vi "Register Status Change Event.vi"() -> ()   [LabVIEW 2017]
doc: "------------- lvcsm -------------\n[CSMStates]\nItem 0 = \"Event Structure\"\nItem 1 = \"Idle\"\nItem 2 = \"CSM Documentation\"\nItem 3 = \"VI Reference\"\nItem 4 = \"Error Handler\"\nItem 5 = \"Critical Error\"\nItem 6 = \"Target Timeout Error\"\nItem 7 = \"Target Error\"\nItem 8 = \"Async Response\"\nItem 9 = \"Response\"\nItem 10 = \"Async Message Posted\"\nItem 11 = \"Initialize Core Data\"\nItem 12 = \"Exit\"\nItem 13 = \"Data: Initialize\"\nItem 14 = \"Data: Cleanup\"\nItem 15 = \"Events: Register\"\nItem 16 = \"Events: Unregister\"\nItem 17 = \"UI: Initialize\"\nItem 18 = \"UI: Cursor Set\"\nItem 19 = \"UI: Front Panel State\"\nItem 20 = \"Macro: Initialize\"\nItem 21 = \"Macro: Exit\"\nItem 22 = \"API: API1\"\nItem 23 = \"API: API2\"\nItem 24 = \"DoSth: DoA\"\nItem 25 = \"DoSth: DoB\"\nItem 26 = \"Handler: Error Occurred\"\n\n[CSMStatus]\nItem 0 = \"Error Occured@\"\nItem 1 = \"Slave Status Changed@\"\nItem 2 = \"Slave Status Changed@\""
uses:
  user.lib/_NEVSTOP/Communicable State Machine(CSM)/AdvanceAPI/CSM - Revert Arguments-Safe String.vi
  user.lib/_NEVSTOP/Communicable State Machine(CSM)/AdvanceAPI/CSM - Break Down Multiple States String.vi
  user.lib/_NEVSTOP/Communicable State Machine(CSM)/AdvanceAPI/CSM - Compact Multiple States.vi
  user.lib/_NEVSTOP/Communicable State Machine(CSM)/AdvanceAPI/CSM - Make String Arguments Safe.vi
  user.lib/_NEVSTOP/Communicable State Machine(CSM)/AdvanceAPI/CSM - Keywords.vi
  user.lib/_NEVSTOP/Communicable State Machine(CSM)/_Shared/Trim Single-line Text.vi
  user.lib/_NEVSTOP/Communicable State Machine(CSM)/_Polymophic/Build Unregister Message.vi
  user.lib/_NEVSTOP/Communicable State Machine(CSM)/_Polymophic/Build Register Message.vi
  user.lib/_NEVSTOP/Communicable State Machine(CSM)/Communicable State Machine.lvlib
panel:
  in  "unregister":bool
  in  "register":bool
  in  "empty":bool
  in  "simulate an error":bool
  in  "Status Change":bool
  out "State History 2":string
  out "State History":string
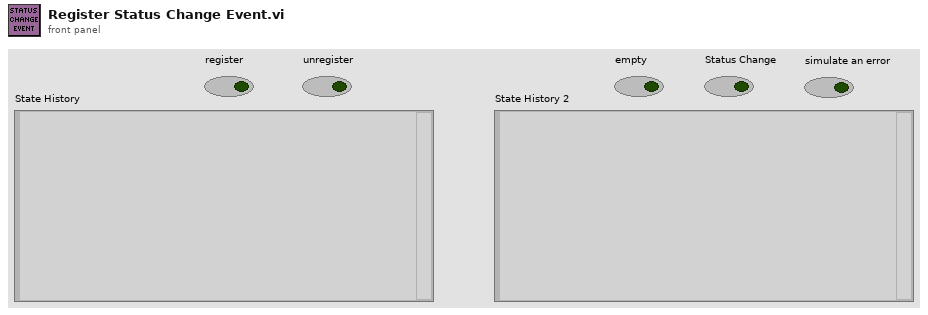
[diagram p1: front panel]
types:
  T1 = enum32{"Invalid", "Standard", "Closed", "Hidden", "Minimized", "Maximized"}
  T2 = enum32{"invalid app kind", "Development System", "Run Time System", "Student Edition", "Embedded LabVIEW", "Evaluation", "Custom"}
  T3 = typedef "Communicable State Machine.lvlib/_CSM_Response Source Message.ctl" = cluster{"‘State":string, "’Arguments":string, "’Error":errorcluster}
  T4 = cluster{"Current VI Reference":refnum<vi>, "Close Panel on Exit?":bool}
  T5 = cluster{"Core":cluster{"Current VI Reference":refnum<vi>, "Close Panel on Exit?":bool}, "Your Boolean data":bool, "Your string data":string}
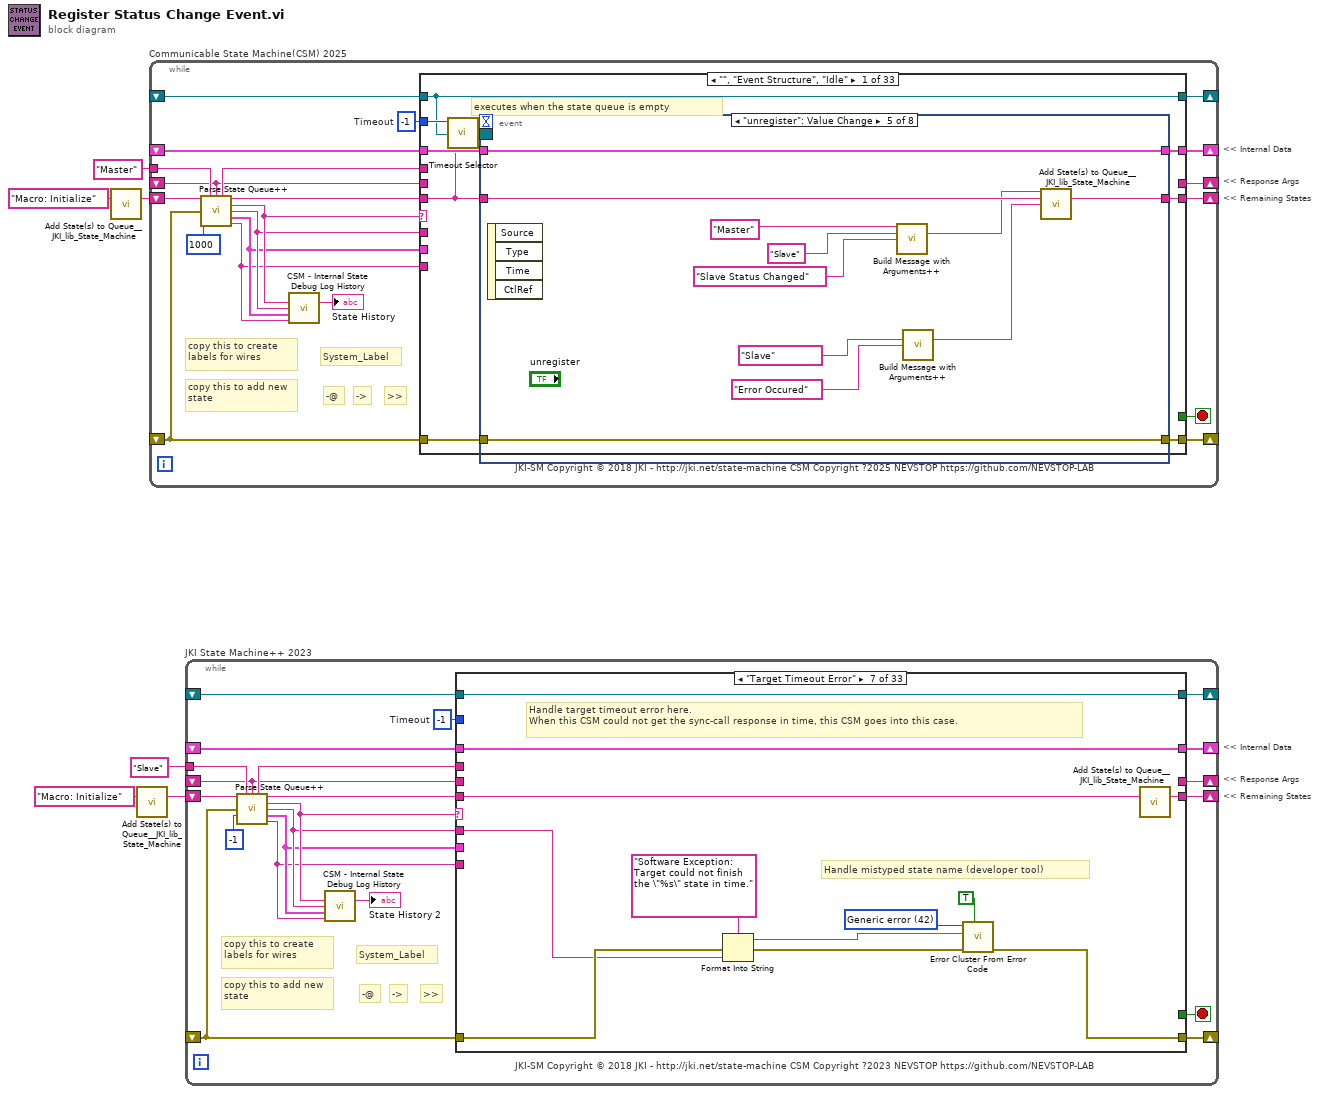
[diagram p0: block diagram]
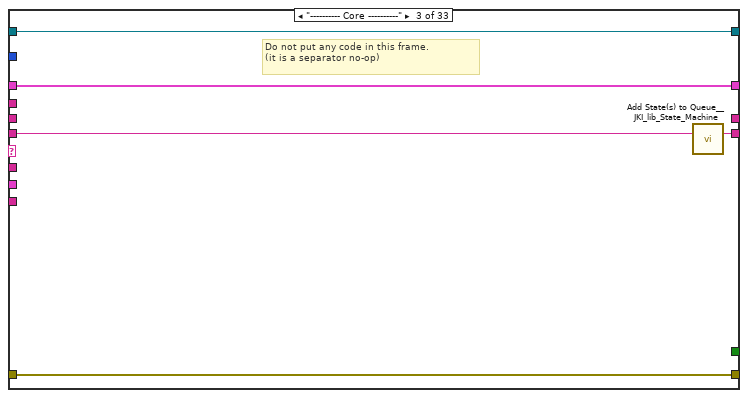
[diagram p4: hidden frame]
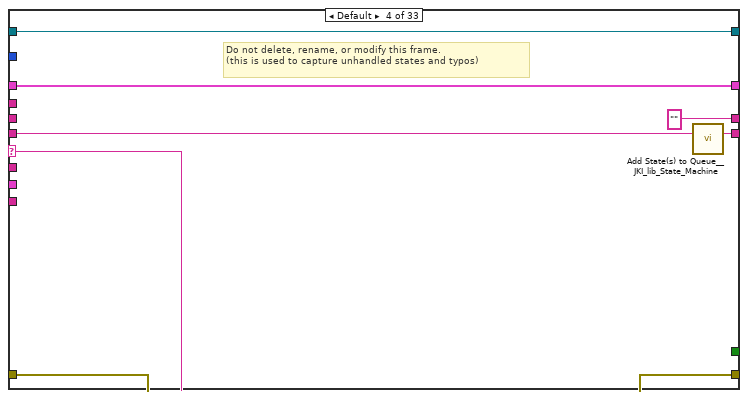
[diagram p5: hidden frame]
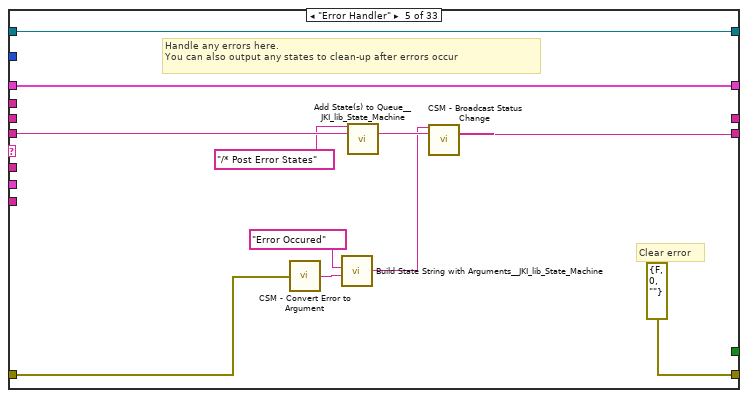
[diagram p6: hidden frame]
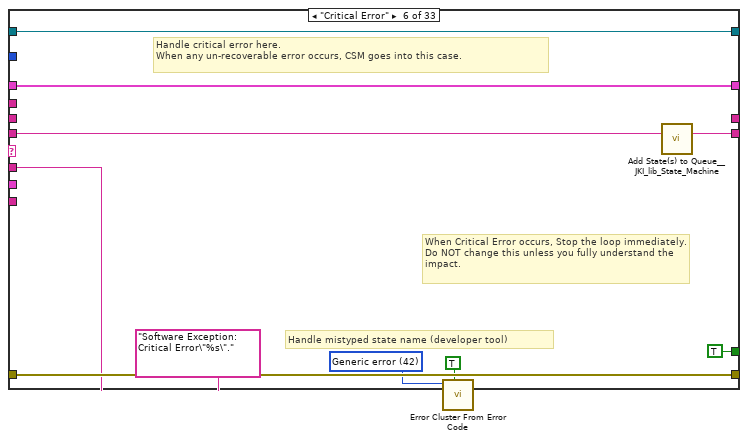
[diagram p7: hidden frame]
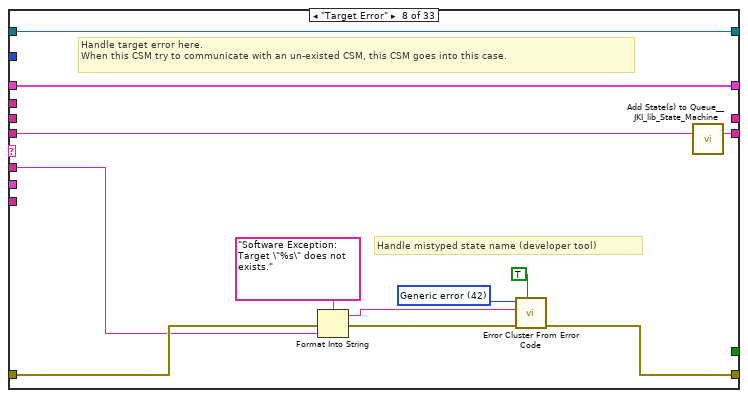
[diagram p8: hidden frame]
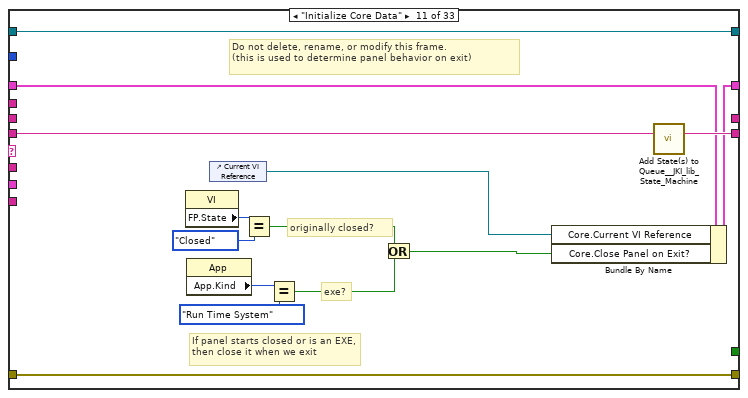
[diagram p11: hidden frame]
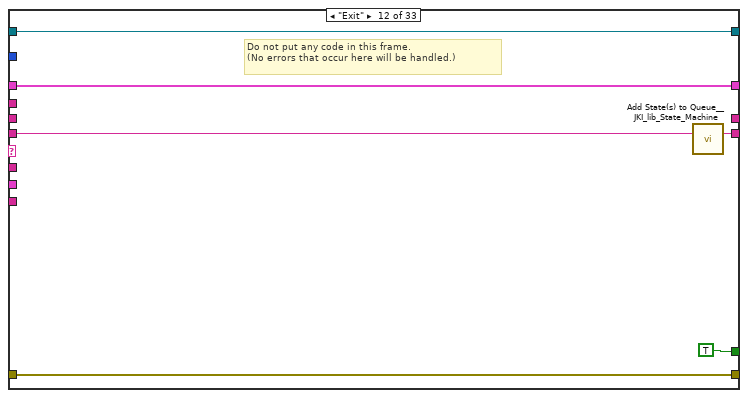
[diagram p12: hidden frame]
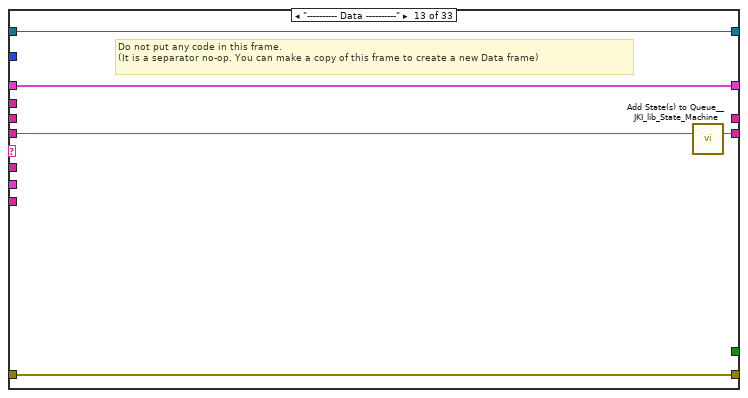
[diagram p13: hidden frame]
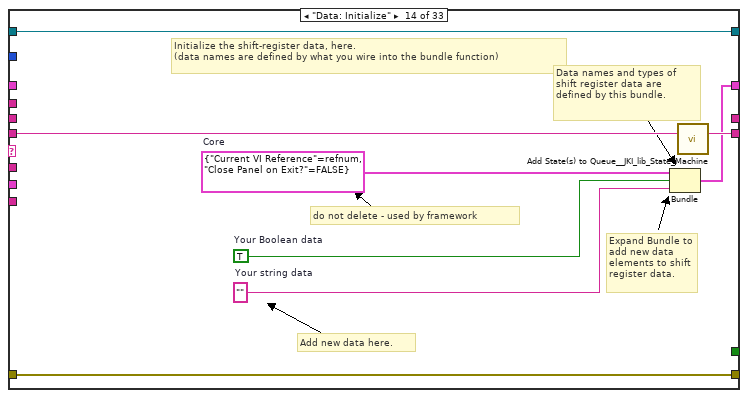
[diagram p14: hidden frame]
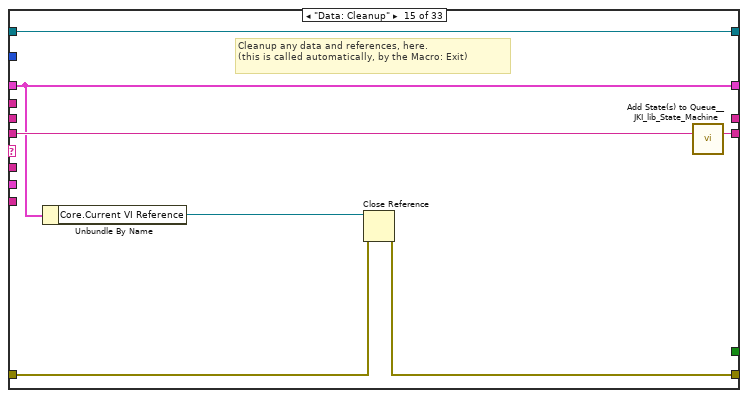
[diagram p15: hidden frame]
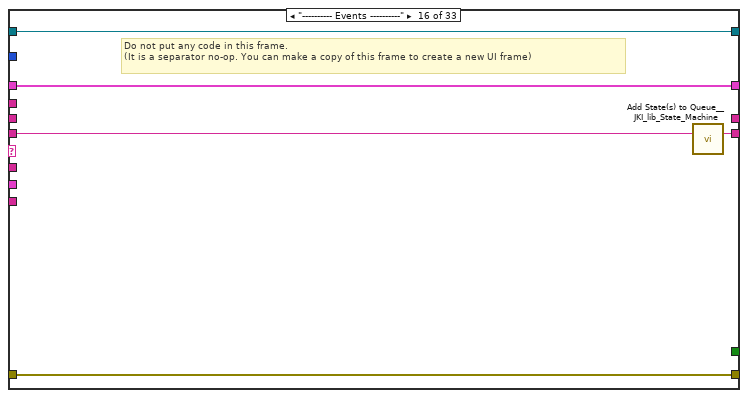
[diagram p16: hidden frame]
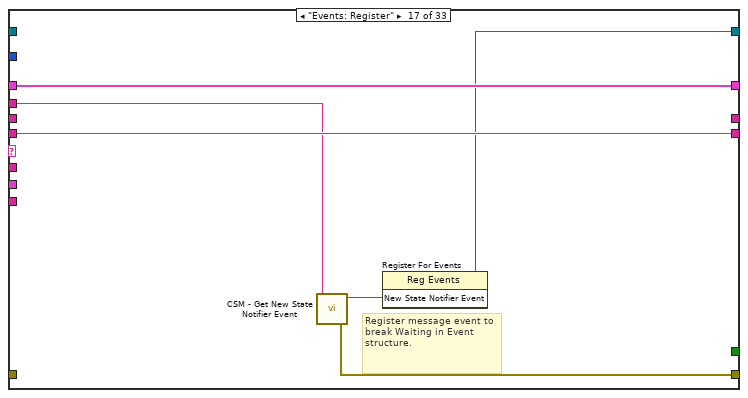
[diagram p17: hidden frame]
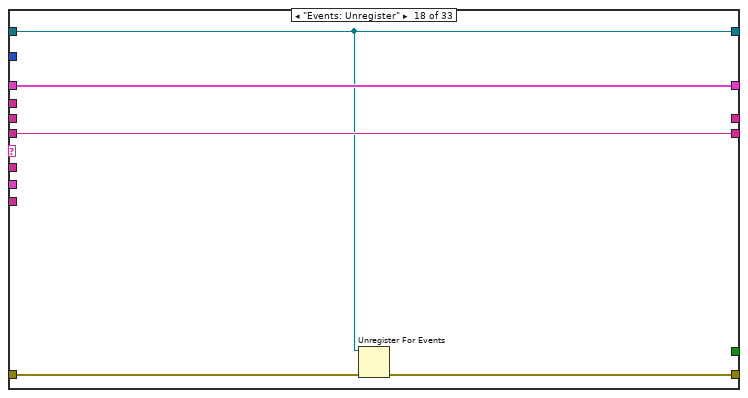
[diagram p18: hidden frame]
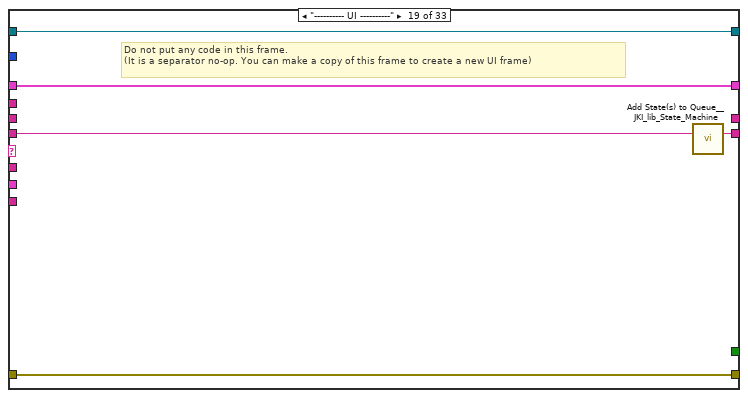
[diagram p19: hidden frame]
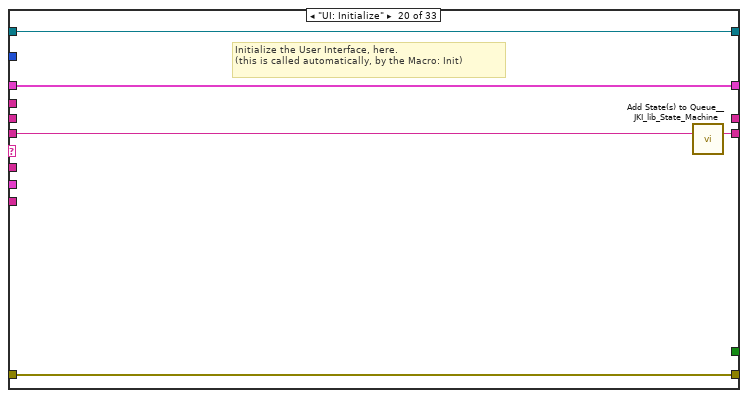
[diagram p20: hidden frame]
diagram:
  # "<< Internal Data"
  # "<< Response Args"
  # "<< Remaining States"
  # "<< Internal Data"
  # "<< Response Args"
  # "<< Remaining States"
  n1 = call <vilib>:"Add State(s) to Queue__JKI_lib_State_Machine.vi"("State(s) in (\"\")"="Macro: Initialize") -> ("States Out"=w6:string)  [unwired: 14 in]
  n2 = call <vilib>:"Add State(s) to Queue__JKI_lib_State_Machine.vi"("State(s) in (\"\")"="Macro: Initialize") -> ("States Out"=w1:string)  [unwired: 14 in]
  n3 = while "Communicable State Machine(CSM) 2025" {
    shift-right: [w22] -> _
    shift-left: _ -> [w21]
    shift-right: [w25] -> _
    shift-left: _ -> [w19]
    shift-right: [w24] -> _
    shift-left: w6 -> [w26]
    tunnel: "Master" ("Name(\"\" to use uuid)") -> [w14]
    shift-right: [w17] -> _
    shift-left: _ -> [w8]
    shift-right: [w16] -> _
    shift-left: _ -> [w15]
    stop <- w23 stop-if-true
    w20 = -1  # Timeout
    # "JKI-SM Copyright © 2018 JKI - http://jki.net/state-machine CSM Copyright ?2025 NEVSTOP https://github.com/NEVSTOP-LAB"
    # "copy this to add new state"
    # ">>"
    # "->"
    # "-@"
    # "copy this to create labels for wires"
    # "System_Label"
    n4 = call "Parse State Queue++.vi"("State Queue"=w26, "Name (\"\" to Use UUID)"=w14, "Response Arguments"=w8, "Previous Error"=w19, "Response Timeout (-2 Use Global Settings)"=1000 ("Response Timeout(1000ms)")) -> ("Name Used"=w9:string, "Remaining States"=w27:string, "Current State"=w13:string, "Arguments"=w12:string, "Additional Information"=w11:T3, "Source CSM"=w10:string)  [unwired: 5 in]
    n5 = call "CSM - Internal State Debug Log History.vi"("State"=w13, "Arguments (\"\")"=w12, ">> Response Source Message >>"=w11, "Source (\"\")"=w10) -> ("Debug Log"=→"State History":string)  [unwired: 11 in]
    n6 = case shown="\"\", \"Event Structure\", \"Idle\"" w13 {
      selector: w13 -> [_ _ _ w97 _ _ _ _ _ _ _ _ _ _ _ _ _ _ _ _ _ _ _ _ _ _ _ _ _ _ _ _ _]
      tunnel: w27 -> [w28 w88 w94 w101 w113 w121 w131 w139 w151 w160 w164 w179 w185 w190 w198 w205 w210 w216 w220 w226 w231 w238 w250 w320 w326 w337 w340 w345 w351 w359 w365 w371 w384]
      tunnel: w12 -> [_ _ _ _ _ _ w124 w135 w147 _ _ _ _ _ _ _ _ _ _ _ _ w233 w244 _ _ _ _ _ w348 _ _ _ w381]
      tunnel: w21 -> [w35 w87 w91 w99 w112 w118 w132 w137 w149 w159 w163 w172 w183 w187 _ w200 w207 w215 w219 w223 w229 w236 w246 w317 w323 w334 w339 w344 w350 w356 w362 w368 w383]
      tunnel: [w34 w89 w92 w103 w114 errorcluster {"status"=FALSE, "code"=0, "source"=""} ("error out") w133 w141 w153 w161 w165 w176 w182 w188 w195 w201 w208 w211 w218 w224 w228 w234 w247 w318 w324 w335 w341 w346 w352 w357 w363 w369 w385] -> w25
      tunnel: w19 -> [w33 w89 w92 w102 w114 w117 w133 w140 w152 w161 w165 w176 w182 w188 w195 w202 w208 _ w221 w224 w228 w235 w248 w318 w324 w335 w341 w346 w352 w357 w363 w369 w385]
      tunnel: [w36 w88 w93 w100 w113 w120 w130 w138 w150 w160 w164 w178 w184 w189 w197 w204 w209 w216 w220 w225 w230 w237 w249 w319 w325 w336 w340 w345 w351 w358 w364 w370 w384] -> w24
      tunnel: [_ _ _ _ _ _ TRUE _ _ _ _ _ TRUE _ _ _ _ _ _ _ _ _ _ _ _ _ _ _ _ _ _ _ _] -> w23
      tunnel: [w32 w87 w91 w99 w112 w118 w132 w137 w149 w159 w163 w177 w183 w187 w196 w200 w207 w215 w219 w223 w229 w236 w246 w317 w323 w334 w339 w344 w350 w356 w362 w368 w383] -> w22
      tunnel: w20 -> [w31 _ _ _ _ _ _ _ _ _ _ _ _ _ _ _ _ _ _ _ _ _ _ _ _ _ _ _ _ _ _ _ _]
      tunnel: w10 -> [_ _ _ _ _ _ _ _ _ _ _ _ _ _ _ _ _ _ _ _ _ _ _ _ _ _ _ _ _ _ _ _ w379]
      tunnel: w11 -> [_ _ _ _ _ _ _ _ _ _ _ _ _ _ _ _ _ _ _ _ _ _ _ _ _ _ _ _ _ _ _ _ w378]
      tunnel: [_ _ _ "" w108 _ _ _ _ _ _ _ _ _ _ _ _ _ _ _ _ _ _ _ _ _ _ "API1 Response" w347 _ "DoA Finished" "DoB Finished" _] -> w17
      tunnel: [w30 w86 w90 w95 w111 w115 w122 w134 w146 w158 w162 w166 w180 w186 w191 w199 w206 w214 w217 w222 w227 w232 w243 w316 w321 w327 w338 w343 w349 w355 w361 w367 w382] -> w16
      tunnel: w15 -> [w30 w86 w90 w95 w111 w115 w122 w134 w146 w158 w162 w166 w180 w186 w191 w199 w206 _ w217 w222 w227 w232 w243 w316 w321 w327 w338 w343 w349 w355 w361 w367 w382]
      tunnel: w9 -> [_ _ _ _ _ _ _ _ _ _ _ _ _ _ _ _ _ w213 _ _ _ _ _ _ _ _ _ _ _ _ _ _ _]
      tunnel: w8 -> [_ _ _ _ _ _ _ _ _ _ _ _ _ _ _ _ _ _ _ _ _ _ _ _ _ _ _ _ _ _ _ _ _]
      frame "", "Event Structure", "Idle" {
        # "executes when the state queue is empty"
        n7 = call "Timeout Selector.vi"("Remaining States"=w28, "Timeout Expected"=w31) -> ("Timeout"=w29:i32)  [unwired: 5 in]
        n8 = event shown="[4] \"unregister\": Value Change" {
          selector: w30 -> [_ _ _ _ _ _ _ _]
          dyn-events: _ -> [_ _ _ _ _ _ _ _]
          timeout: w29 -> [_ _ _ _ _ _ _ _]
          tunnel: w28 -> [w40 w43 w46 w58 w69 w73 w80 w85]
          tunnel: [w39 w43 w45 w57 w68 w73 w79 w85] -> w36
          tunnel: w35 -> [w37 w41 w47 w59 w70 w74 w77 w83]
          tunnel: [w38 w42 w48 w60 w71 w72 w78 w84] -> w34
          tunnel: w33 -> [w38 w42 w48 w60 w71 w72 w78 w84]
          tunnel: [w37 w41 w47 w59 w70 w74 w77 w83] -> w32
          event Timeout {
            n9 = event-data() -> ()  [unwired: 1 in, 1 out]
            n10 = call <vilib>:"Add State(s) to Queue__JKI_lib_State_Machine.vi"("State(s) in (\"\")"=w40) -> ("States Out"=w39:string)  [unwired: 14 in]
          }
          event "empty": Value Change {
            n11 = event-data() -> ()  [unwired: 1 in, 4 out]
          }
          event "simulate an error": Value Change {
            n12 = event-data() -> ()  [unwired: 1 in, 4 out]
            n13 = call <vilib>:"Add State(s) to Queue__JKI_lib_State_Machine.vi"("State(s) in Front (\"\")"="simulate an error ->| Slave" ("State(s) in Front (\"\")"), "State(s) in (\"\")"=w46) -> ("States Out"=w45:string)  [unwired: 13 in]
          }
          event "register": Value Change {
            n14 = event-data() -> ()  [unwired: 1 in, 4 out]
            n15 = call-poly "Build Message with Arguments++.vi"("Source CSM (* as Default)"="Slave" ("Name(\"\" to use uuid)"), "Status"="Slave Status Changed" ("Message"), "API (If \"\", Same As \"Status\")"="DoSth: DoA" ("Response Message (\"\" to use Message)")) -> ("CSM Message String"=w53:string)  [unwired: 12 in]
            n16 = call-poly "Build Message with Arguments++.vi"("Source CSM (* as Default)"="Slave" ("Name(\"\" to use uuid)"), "Status"="Error Occured" ("Message"), "API (If \"\", Same As \"Status\")"="Handler: Error Occurred" ("Response Message (\"\" to use Message)")) -> ("CSM Message String"=w49:string)  [unwired: 12 in]
            n17 = call <vilib>:"Add State(s) to Queue__JKI_lib_State_Machine.vi"("State(s) in Front (\"\")"=w53, "State(s) in (\"\")"=w58, "State(s) at Back (\"\")"=w49) -> ("States Out"=w57:string)  [unwired: 12 in]
          }
          event "unregister": Value Change {
            n18 = event-data() -> ()  [unwired: 1 in, 4 out]
            n19 = call-poly "Build Message with Arguments++.vi"("Target CSM"="Master" ("Source CSM Name"), "Source CSM (* as Default)"="Slave" ("Name(\"\" to use uuid)"), "Status"="Slave Status Changed" ("Message")) -> ("CSM Message String"=w64:string)  [unwired: 12 in]
            n20 = call-poly "Build Message with Arguments++.vi"("Source CSM (* as Default)"="Slave" ("Name(\"\" to use uuid)"), "Status"="Error Occured" ("Message")) -> ("CSM Message String"=w61:string)  [unwired: 13 in]
            n21 = call <vilib>:"Add State(s) to Queue__JKI_lib_State_Machine.vi"("State(s) in Front (\"\")"=w64, "State(s) in (\"\")"=w69, "State(s) at Back (\"\")"=w61) -> ("States Out"=w68:string)  [unwired: 12 in]
          }
          event User Event {
            # "This user event is used to break out CSM from waiting in the event structure, to process the next state from external. DO NOT place any code here unless you really need to."
            n22 = event-data() -> ()  [unwired: 1 in, 1 out]
          }
          event Panel Close? {
            # "Discard the event because we'll close the front panel ourselves in Macro: Exit"
            # "Close Panel button (pressed) Event\n(this executes Macro: Exit to terminate the VI)"
            n23 = event-data() -> ()  [unwired: 1 in, 1 out]
            n24 = event-data("Discard?"=TRUE) -> ()  [unwired: 1 in, 1 out]
            n25 = call <vilib>:"Add State(s) to Queue__JKI_lib_State_Machine.vi"("State(s) in Front (\"\")"="Macro: Exit -@ Slave\nMacro: Exit", "State(s) in (\"\")"=w80) -> ("States Out"=w79:string)  [unwired: 13 in]
          }
          event "Status Change": Value Change {
            n26 = event-data() -> ()  [unwired: 1 in, 6 out]
            n27 = call "CSM - Post Message.vi"("Target Module"="Slave" ("Dest Module"), "State"="Status Change" ("States")) -> ()  [unwired: 9 in, 1 out]
          }
        }
      }
      frame "CSM Documentation" {
        # "CSM Documentation"
        # "State Syntax:\nStateCategory: State >> Argument @|-> CSMName\nLine Terminator: Line feed\n\nExample:\nUI: Help >> About @Main\nUI: Help >> About ->Main"
        # "Commenting:\nTo add a comment use \"//\" or \"#\" and all text to the right will be ignored\nCommenting Example:\nUI: Initialize // This initializes the UI\n# This whole line is a comment\n// Another comment line"
      }
      frame "---------- Core ----------" {
        # "Do not put any code in this frame.\n(it is a separator no-op)"
        n28 = call <vilib>:"Add State(s) to Queue__JKI_lib_State_Machine.vi"("State(s) in (\"\")"=w94) -> ("States Out"=w93:string)  [unwired: 14 in]
      }
      frame Default {
        w106 = 42 items=["No error", "Argument error", "Memory is full", "Out of zone", "End of file", "File already open", "Generic file I/O error", "File not found", "File permission error", "Disk is full", "Duplicate path", "Too many files open", "System feature not enabled", "Resource file not found", "Cannot add resource", "Resource not found", "Image not found", "Image memory error", "Pen does not exist", "Config type invalid", "Config token not found", "Config parse error", "Config memory error", "Bad external code format", "Bad external code offset", "External code not present", "Null window", "Destroy window error", "Null menu", "Print aborted", "Bad print record", "Print driver error", "Windows error during printing", "Memory error during printing", "Print dialog error", "Generic print error", "Invalid device refnum", "Device not found", "Device parameter error", "Device unit error", "Cannot open device", "Device call aborted", "Generic error", "Cancelled by user", "Object ID too low", "Object ID too high", "Object not in heap", "Unknown heap", "Unknown object (invalid DefProc)", "Unknown object (DefProc not in table)", "Message out of range", "Invalid (null) method", "Unknown message", "Manager call not supported", "Bad address", "Network operation in progress", "Network operation timed out", "Connection is busy", "Network attribute not supported", "Network error", "Address in use", "System out of memory", "Connection aborted", "Connection refused", "Not connected", "Already connected", "Connection closed", "Initialization error (interapplication manager)", "Bad occurrence", "Wait on unbound occurrence handler", "Occurrence queue overflow", "Datalog type conflict", "Unused", "Unrecognized type (interapplication manager)", "Memory corrupt", "Failed to make temporary DLL", "Old CIN version", "Drag socket not found", "Failed to load drop-object", "Failed to register OLE object", "Failed to release OLE object", "Format specifier type mismatch", "Unknown format specifier", "Too few format specifiers", "Too many format specifiers", "Scan failed", "Newer CIN version", "Error converting to variant", "Runtime menu error", "Password tampered", "Variant attribute not found", "Incompatible variant data type", "Event data is not available", "Event Store is not present", "Occurrence is not found", "Event Queue is not created", "Event info is not available", "Refnum passed is NULL", "Error retrieving Class GUID", "Error retrieving CoClass GUID", "Error retrieving TypeLib GUID.", "Bad built application magic bytes.", "Specific driver is different from the specific driver associated with the Logical Name.", "There is no session opened to the class driver.", "Max Error", "MAX - Error with config objects", "MAX - Error loading configuration", "MAX - Group not supported"]
        # "Do not delete, rename, or modify this frame.\n(this is used to capture unhandled states and typos)"
        # "Handle mistyped state name (developer tool)"
        n29 = Format Into String(format string="Software Exception: Unhandled State \"%s\"." ("message"), error in=w102, w97) -> (resulting string=w105:string, error out=w104:errorcluster)  [unwired: 1 in]
        n30 = call <vilib>:"Error Cluster From Error Code.vi"("show call chain? (False)"=TRUE, "error in (no error)"=w104, "error message (\"\")"=w105, "error code (0)"=w106) -> ("error out"=w103:errorcluster)  [unwired: 5 in]
        n31 = call <vilib>:"Add State(s) to Queue__JKI_lib_State_Machine.vi"("State(s) in (\"\")"=w101) -> ("States Out"=w100:string)  [unwired: 14 in]
      }
      frame "VI Reference" {
        n32 = Unbundle By Name(w112) -> ("Core"=w110:T4)
        n33 = Unbundle By Name(w110) -> ("Current VI Reference"=w109:refnum<vi>)
        n34 = call "CSM - Convert Data to HexStr.vi"("Variant"=w109) -> ("HEX String (0-9,A-F)"=w108:string)  [unwired: 8 in]
      }
      frame "Error Handler" {
        # "Unhandled Error -- Display it"
        # "Handle any errors here.\nYou can also output any states to clean-up after errors occur"
        # "Clear error"
        n35 = call <vilib>:"General Error Handler.vi"("error in (no error)"=w117) -> ()  [unwired: 10 in, 5 out]
        n36 = call <vilib>:"Add State(s) to Queue__JKI_lib_State_Machine.vi"("State(s) in Front (\"\")"="/* Post Error States", "State(s) in (\"\")"=w121) -> ("States Out"=w120:string)  [unwired: 13 in]
      }
      frame "Critical Error" {
        w128 = 42 items=["No error", "Argument error", "Memory is full", "Out of zone", "End of file", "File already open", "Generic file I/O error", "File not found", "File permission error", "Disk is full", "Duplicate path", "Too many files open", "System feature not enabled", "Resource file not found", "Cannot add resource", "Resource not found", "Image not found", "Image memory error", "Pen does not exist", "Config type invalid", "Config token not found", "Config parse error", "Config memory error", "Bad external code format", "Bad external code offset", "External code not present", "Null window", "Destroy window error", "Null menu", "Print aborted", "Bad print record", "Print driver error", "Windows error during printing", "Memory error during printing", "Print dialog error", "Generic print error", "Invalid device refnum", "Device not found", "Device parameter error", "Device unit error", "Cannot open device", "Device call aborted", "Generic error", "Cancelled by user", "Object ID too low", "Object ID too high", "Object not in heap", "Unknown heap", "Unknown object (invalid DefProc)", "Unknown object (DefProc not in table)", "Message out of range", "Invalid (null) method", "Unknown message", "Manager call not supported", "Bad address", "Network operation in progress", "Network operation timed out", "Connection is busy", "Network attribute not supported", "Network error", "Address in use", "System out of memory", "Connection aborted", "Connection refused", "Not connected", "Already connected", "Connection closed", "Initialization error (interapplication manager)", "Bad occurrence", "Wait on unbound occurrence handler", "Occurrence queue overflow", "Datalog type conflict", "Unused", "Unrecognized type (interapplication manager)", "Memory corrupt", "Failed to make temporary DLL", "Old CIN version", "Drag socket not found", "Failed to load drop-object", "Failed to register OLE object", "Failed to release OLE object", "Format specifier type mismatch", "Unknown format specifier", "Too few format specifiers", "Too many format specifiers", "Scan failed", "Newer CIN version", "Error converting to variant", "Runtime menu error", "Password tampered", "Variant attribute not found", "Incompatible variant data type", "Event data is not available", "Event Store is not present", "Occurrence is not found", "Event Queue is not created", "Event info is not available", "Refnum passed is NULL", "Error retrieving Class GUID", "Error retrieving CoClass GUID", "Error retrieving TypeLib GUID.", "Bad built application magic bytes.", "Specific driver is different from the specific driver associated with the Logical Name.", "There is no session opened to the class driver.", "Max Error", "MAX - Error with config objects", "MAX - Error loading configuration", "MAX - Group not supported"]
        # "Handle critical error here.\nWhen any un-recoverable error occurs, CSM goes into this case."
        # "When Critical Error occurs, Stop the loop immediately. Do NOT change this unless you fully understand the impact."
        # "Handle mistyped state name (developer tool)"
        n37 = Format Into String(format string="Software Exception: Critical Error\"%s\"." ("message"), w124) -> (resulting string=w127:string, error out=w126:errorcluster)  [unwired: 2 in]
        n38 = call <vilib>:"Error Cluster From Error Code.vi"("show call chain? (False)"=TRUE, "error in (no error)"=w126, "error message (\"\")"=w127, "error code (0)"=w128) -> ()  [unwired: 5 in, 1 out]
        n39 = call <vilib>:"Add State(s) to Queue__JKI_lib_State_Machine.vi"("State(s) in (\"\")"=w131) -> ("States Out"=w130:string)  [unwired: 14 in]
      }
      frame "Target Timeout Error" {
        w144 = 42 items=["No error", "Argument error", "Memory is full", "Out of zone", "End of file", "File already open", "Generic file I/O error", "File not found", "File permission error", "Disk is full", "Duplicate path", "Too many files open", "System feature not enabled", "Resource file not found", "Cannot add resource", "Resource not found", "Image not found", "Image memory error", "Pen does not exist", "Config type invalid", "Config token not found", "Config parse error", "Config memory error", "Bad external code format", "Bad external code offset", "External code not present", "Null window", "Destroy window error", "Null menu", "Print aborted", "Bad print record", "Print driver error", "Windows error during printing", "Memory error during printing", "Print dialog error", "Generic print error", "Invalid device refnum", "Device not found", "Device parameter error", "Device unit error", "Cannot open device", "Device call aborted", "Generic error", "Cancelled by user", "Object ID too low", "Object ID too high", "Object not in heap", "Unknown heap", "Unknown object (invalid DefProc)", "Unknown object (DefProc not in table)", "Message out of range", "Invalid (null) method", "Unknown message", "Manager call not supported", "Bad address", "Network operation in progress", "Network operation timed out", "Connection is busy", "Network attribute not supported", "Network error", "Address in use", "System out of memory", "Connection aborted", "Connection refused", "Not connected", "Already connected", "Connection closed", "Initialization error (interapplication manager)", "Bad occurrence", "Wait on unbound occurrence handler", "Occurrence queue overflow", "Datalog type conflict", "Unused", "Unrecognized type (interapplication manager)", "Memory corrupt", "Failed to make temporary DLL", "Old CIN version", "Drag socket not found", "Failed to load drop-object", "Failed to register OLE object", "Failed to release OLE object", "Format specifier type mismatch", "Unknown format specifier", "Too few format specifiers", "Too many format specifiers", "Scan failed", "Newer CIN version", "Error converting to variant", "Runtime menu error", "Password tampered", "Variant attribute not found", "Incompatible variant data type", "Event data is not available", "Event Store is not present", "Occurrence is not found", "Event Queue is not created", "Event info is not available", "Refnum passed is NULL", "Error retrieving Class GUID", "Error retrieving CoClass GUID", "Error retrieving TypeLib GUID.", "Bad built application magic bytes.", "Specific driver is different from the specific driver associated with the Logical Name.", "There is no session opened to the class driver.", "Max Error", "MAX - Error with config objects", "MAX - Error loading configuration", "MAX - Group not supported"]
        # "Handle target timeout error here.\nWhen this CSM could not get the sync-call response in time, this CSM goes into this case."
        # "Handle mistyped state name (developer tool)"
        n40 = Format Into String(format string="Software Exception: Target could not finish the \"%s\" state in time." ("message"), error in=w140, w135) -> (resulting string=w143:string, error out=w142:errorcluster)  [unwired: 1 in]
        n41 = call <vilib>:"Error Cluster From Error Code.vi"("show call chain? (False)"=TRUE, "error in (no error)"=w142, "error message (\"\")"=w143, "error code (0)"=w144) -> ("error out"=w141:errorcluster)  [unwired: 5 in]
        n42 = call <vilib>:"Add State(s) to Queue__JKI_lib_State_Machine.vi"("State(s) in (\"\")"=w139) -> ("States Out"=w138:string)  [unwired: 14 in]
      }
      frame "Target Error" {
        w156 = 42 items=["No error", "Argument error", "Memory is full", "Out of zone", "End of file", "File already open", "Generic file I/O error", "File not found", "File permission error", "Disk is full", "Duplicate path", "Too many files open", "System feature not enabled", "Resource file not found", "Cannot add resource", "Resource not found", "Image not found", "Image memory error", "Pen does not exist", "Config type invalid", "Config token not found", "Config parse error", "Config memory error", "Bad external code format", "Bad external code offset", "External code not present", "Null window", "Destroy window error", "Null menu", "Print aborted", "Bad print record", "Print driver error", "Windows error during printing", "Memory error during printing", "Print dialog error", "Generic print error", "Invalid device refnum", "Device not found", "Device parameter error", "Device unit error", "Cannot open device", "Device call aborted", "Generic error", "Cancelled by user", "Object ID too low", "Object ID too high", "Object not in heap", "Unknown heap", "Unknown object (invalid DefProc)", "Unknown object (DefProc not in table)", "Message out of range", "Invalid (null) method", "Unknown message", "Manager call not supported", "Bad address", "Network operation in progress", "Network operation timed out", "Connection is busy", "Network attribute not supported", "Network error", "Address in use", "System out of memory", "Connection aborted", "Connection refused", "Not connected", "Already connected", "Connection closed", "Initialization error (interapplication manager)", "Bad occurrence", "Wait on unbound occurrence handler", "Occurrence queue overflow", "Datalog type conflict", "Unused", "Unrecognized type (interapplication manager)", "Memory corrupt", "Failed to make temporary DLL", "Old CIN version", "Drag socket not found", "Failed to load drop-object", "Failed to register OLE object", "Failed to release OLE object", "Format specifier type mismatch", "Unknown format specifier", "Too few format specifiers", "Too many format specifiers", "Scan failed", "Newer CIN version", "Error converting to variant", "Runtime menu error", "Password tampered", "Variant attribute not found", "Incompatible variant data type", "Event data is not available", "Event Store is not present", "Occurrence is not found", "Event Queue is not created", "Event info is not available", "Refnum passed is NULL", "Error retrieving Class GUID", "Error retrieving CoClass GUID", "Error retrieving TypeLib GUID.", "Bad built application magic bytes.", "Specific driver is different from the specific driver associated with the Logical Name.", "There is no session opened to the class driver.", "Max Error", "MAX - Error with config objects", "MAX - Error loading configuration", "MAX - Group not supported"]
        # "Handle target error here.\nWhen this CSM try to communicate with an un-existed CSM, this CSM goes into this case."
        # "Handle mistyped state name (developer tool)"
        n43 = Format Into String(format string="Software Exception: Target \"%s\" does not exists." ("message"), error in=w152, w147) -> (resulting string=w155:string, error out=w154:errorcluster)  [unwired: 1 in]
        n44 = call <vilib>:"Error Cluster From Error Code.vi"("show call chain? (False)"=TRUE, "error in (no error)"=w154, "error message (\"\")"=w155, "error code (0)"=w156) -> ("error out"=w153:errorcluster)  [unwired: 5 in]
        n45 = call <vilib>:"Add State(s) to Queue__JKI_lib_State_Machine.vi"("State(s) in (\"\")"=w151) -> ("States Out"=w150:string)  [unwired: 14 in]
      }
      frame "Async Response", "Response" {
        # "Handle Async-call Response (\"Async Response\" for ->)"
        # "Handle Sync-call Response (\"Response\" for @)"
        # "After Message is executed, CSM goes to this state for receive the response. \n    For Async Message(->), \"Async Response\" is used. This CSM will goes to \"Async Message Posted\" immediately and receive the \"Async Response\" after the callee finishes the message.\n    For Sync Message(@),  This CSM will wait until the message is done and immediately goes to \"Response\""
      }
      frame "Async Message Posted" {
        # "Handle post action for async message (->)."
        # "After Async Message is posted (->), CSM goes to this state for post-action. You can use Argument - State to tell which Async Message is called."
      }
      frame "Initialize Core Data" {
        # "Do not delete, rename, or modify this frame.\n(this is used to determine panel behavior on exit)"
        # "originally closed?"
        # "exe?"
        # "If panel starts closed or is an EXE, then close it when we exit"
        n46 = property class="VI"() -> ("FP.State"=w169:T1)  [unwired: 2 in, 2 out]
        n47 = property class="App"() -> ("App.Kind"=w175:T2)  [unwired: 2 in, 2 out]
        n48 = control-ref of="Current VI Reference"() -> (w170:refnum<vi>)
        n49 = Equal?(x=w169, y=T1."Closed" ("Front Panel Window:State")) -> (x = y?=w167:bool)
        n50 = Equal?(x=w175, y=T2."Run Time System" ("Application:Kind")) -> (x = y?=w173:bool)
        n51 = Or(x=w167, y=w173) -> (x .or. y?=w171:bool)
        n52 = Bundle By Name(cluster=w172, "Core.Current VI Reference"=w170, "Core.Close Panel on Exit?"=w171) -> (w177:T5)
        n53 = call <vilib>:"Add State(s) to Queue__JKI_lib_State_Machine.vi"("State(s) in (\"\")"=w179) -> ("States Out"=w178:string)  [unwired: 14 in]
      }
      frame "Exit" {
        # "Do not put any code in this frame.\n(No errors that occur here will be handled.)"
        n54 = call <vilib>:"Add State(s) to Queue__JKI_lib_State_Machine.vi"("State(s) in (\"\")"=w185) -> ("States Out"=w184:string)  [unwired: 14 in]
      }
      frame "---------- Data ----------" {
        # "Do not put any code in this frame.\n(It is a separator no-op. You can make a copy of this frame to create a new Data frame)"
        n55 = call <vilib>:"Add State(s) to Queue__JKI_lib_State_Machine.vi"("State(s) in (\"\")"=w190) -> ("States Out"=w189:string)  [unwired: 14 in]
      }
      frame "Data: Initialize" {
        w192 = T4 {"Current VI Reference"=refnum, "Close Panel on Exit?"=FALSE}  # Core
        w194 = TRUE  # Your Boolean data
        w193 = ""  # Your string data
        # "do not delete - used by framework"
        # "Expand Bundle to add new data elements to shift register data."
        # "Add new data here."
        # "Data names and types of shift register data are defined by this bundle."
        # "Initialize the shift-register data, here.\n(data names are defined by what you wire into the bundle function)"
        n56 = Bundle("Core"=w192, "Your Boolean data"=w194, "Your string data"=w193) -> (w196:T5)  [unwired: 1 in]
        n57 = call <vilib>:"Add State(s) to Queue__JKI_lib_State_Machine.vi"("State(s) in (\"\")"=w198) -> ("States Out"=w197:string)  [unwired: 14 in]
      }
      frame "Data: Cleanup" {
        # "Cleanup any data and references, here.\n(this is called automatically, by the Macro: Exit)"
        n58 = Unbundle By Name(w200) -> ("Core.Current VI Reference"=w203:refnum<vi>)
        n59 = Close Reference(reference=w203, error in (no error)=w202) -> (error out=w201:errorcluster)
        n60 = call <vilib>:"Add State(s) to Queue__JKI_lib_State_Machine.vi"("State(s) in (\"\")"=w205) -> ("States Out"=w204:string)  [unwired: 14 in]
      }
      frame "---------- Events ----------" {
        # "Do not put any code in this frame.\n(It is a separator no-op. You can make a copy of this frame to create a new UI frame)"
        n61 = call <vilib>:"Add State(s) to Queue__JKI_lib_State_Machine.vi"("State(s) in (\"\")"=w210) -> ("States Out"=w209:string)  [unwired: 14 in]
      }
      frame "Events: Register" {
        # "Register message event to break Waiting in Event structure."
        n62 = call "CSM - Get New State Notifier Event.vi"("Name (\"\" to Use UUID)"=w213) -> ("error out"=w211:errorcluster, "New State Notifier Event"=w212:refnum<user-event>)  [unwired: 9 in]
        n63 = register-events(w212) -> (reference out=w214:refnum<event-registration>)  [unwired: 2 in, 1 out]
      }
      frame "Events: Unregister" {
        n64 = Unregister For Events(event registration refnum=w217, error in=w221) -> (error out=w218:errorcluster)
      }
      frame "---------- UI ----------" {
        # "Do not put any code in this frame.\n(It is a separator no-op. You can make a copy of this frame to create a new UI frame)"
        n65 = call <vilib>:"Add State(s) to Queue__JKI_lib_State_Machine.vi"("State(s) in (\"\")"=w226) -> ("States Out"=w225:string)  [unwired: 14 in]
      }
      frame "UI: Initialize" {
        # "Initialize the User Interface, here.\n(this is called automatically, by the Macro: Init)"
        n66 = call <vilib>:"Add State(s) to Queue__JKI_lib_State_Machine.vi"("State(s) in (\"\")"=w231) -> ("States Out"=w230:string)  [unwired: 14 in]
      }
      frame "UI: Cursor Set" {
        # "Argument"
        # "Set and Unset Cursor Busy.\n(Usage: \"UI: Cursor Set >> Busy|Idle\")"
        n67 = case shown="\"Idle\", Default" w233 {
          tunnel: w235 -> [w240 w242]
          tunnel: [w239 w241] -> w234
          frame "Idle", Default {
            n68 = call <vilib>:"Unset Busy.vi"("error in (no error)"=w240) -> ("error out"=w239:errorcluster)  [unwired: 10 in]
          }
          frame "Busy" {
            n69 = call <vilib>:"Set Busy.vi"("error in (no error)"=w242) -> ("error out"=w241:errorcluster)  [unwired: 9 in, 1 out]
          }
        }
        n70 = call <vilib>:"Add State(s) to Queue__JKI_lib_State_Machine.vi"("State(s) in (\"\")"=w238) -> ("States Out"=w237:string)  [unwired: 14 in]
      }
      frame "UI: Front Panel State" {
        # "Argument"
        # "Set Front Panel Open or Closed\n(Usage: \"UI: Front Panel State >> Open|Close\")"
        n71 = Unbundle By Name(w246) -> ("Core.Current VI Reference"=w245:refnum<vi>)
        n72 = case shown="\"Minimize\", \"Minimized\"" w244 {
          tunnel: w248 -> [w256 w271 w282 w295 w308]
          tunnel: [w258 w272 w284 w297 w310] -> w247
          tunnel: w245 -> [w257 w269 w283 w296 w309]
          frame "Open", "Standard", Default {
            w251 = T1."Standard" ("State")
            n73 = property class="VI"(reference=w257, error in=w256) -> (reference out=w254:refnum<vi>, error out=w255:errorcluster, "FP.State"=w253:T1)
            n74 = Not Equal?(x=w253, y=w251) -> (x != y?=w252:bool)
            n75 = case shown="True" w252 {
              tunnel: [w262 w264] -> w258
              tunnel: w255 -> [w261 w264]
              tunnel: w254 -> [w260 _]
              tunnel: w251 -> [w259 _]
              frame True {
                n76 = invoke class="VI" method="FP.Open"(reference=w260, error in=w261, "Activate"=TRUE, "State"=w259) -> (error out=w262:errorcluster)  [unwired: 1 in, 4 out]
              }
              frame False {
              }
            }
          }
          frame "Close", "Closed" {
            n77 = property class="VI"(reference=w269, error in=w271) -> (reference out=w268:refnum<vi>, error out=w270:errorcluster, "FP.State"=w266:T1)
            n78 = Not Equal?(x=w266, y=T1."Closed" ("Front Panel Window:State")) -> (x != y?=w265:bool)
            n79 = case shown="True" w265 {
              tunnel: [w273 w276] -> w272
              tunnel: w270 -> [w273 w275]
              tunnel: w268 -> [_ w274]
              frame False {
              }
              frame True {
                n80 = invoke class="VI" method="FP.Close"(reference=w274, error in=w275) -> (error out=w276:errorcluster)  [unwired: 1 in, 2 out]
              }
            }
          }
          frame "Hidden", "Hide" {
            w277 = T1."Hidden" ("State")
            n81 = property class="VI"(reference=w283, error in=w282) -> (reference out=w280:refnum<vi>, error out=w281:errorcluster, "FP.State"=w279:T1)
            n82 = Not Equal?(x=w279, y=w277) -> (x != y?=w278:bool)
            n83 = case shown="True" w278 {
              tunnel: [w288 w289] -> w284
              tunnel: w281 -> [w287 w289]
              tunnel: w280 -> [w286 _]
              tunnel: w277 -> [w285 _]
              frame True {
                n84 = invoke class="VI" method="FP.Open"(reference=w286, error in=w287, "State"=w285) -> (error out=w288:errorcluster)  [unwired: 2 in, 4 out]
              }
              frame False {
              }
            }
          }
          frame "Minimize", "Minimized" {
            w290 = T1."Minimized" ("State")
            n85 = property class="VI"(reference=w296, error in=w295) -> (reference out=w293:refnum<vi>, error out=w294:errorcluster, "FP.State"=w292:T1)
            n86 = Not Equal?(x=w292, y=w290) -> (x != y?=w291:bool)
            n87 = case shown="True" w291 {
              tunnel: [w301 w302] -> w297
              tunnel: w294 -> [w300 w302]
              tunnel: w293 -> [w299 _]
              tunnel: w290 -> [w298 _]
              frame True {
                n88 = invoke class="VI" method="FP.Open"(reference=w299, error in=w300, "State"=w298) -> (error out=w301:errorcluster)  [unwired: 2 in, 4 out]
              }
              frame False {
              }
            }
          }
          frame "Maximize", "Maximized" {
            w303 = T1."Maximized" ("State")
            n89 = property class="VI"(reference=w309, error in=w308) -> (reference out=w306:refnum<vi>, error out=w307:errorcluster, "FP.State"=w305:T1)
            n90 = Not Equal?(x=w305, y=w303) -> (x != y?=w304:bool)
            n91 = case shown="True" w304 {
              tunnel: [w314 w315] -> w310
              tunnel: w307 -> [w313 w315]
              tunnel: w306 -> [w312 _]
              tunnel: w303 -> [w311 _]
              frame True {
                n92 = invoke class="VI" method="FP.Open"(reference=w312, error in=w313, "State"=w311) -> (error out=w314:errorcluster)  [unwired: 2 in, 4 out]
              }
              frame False {
              }
            }
          }
        }
        n93 = call <vilib>:"Add State(s) to Queue__JKI_lib_State_Machine.vi"("State(s) in (\"\")"=w250) -> ("States Out"=w249:string)  [unwired: 14 in]
      }
      frame "---------- Macro ----------" {
        # "Do not put any code in this frame.\n(It is a separator no-op. You can make a copy of this frame to create a new Macro frame)"
        n94 = call <vilib>:"Add State(s) to Queue__JKI_lib_State_Machine.vi"("State(s) in (\"\")"=w320) -> ("States Out"=w319:string)  [unwired: 14 in]
      }
      frame "Macro: Initialize" {
        w322 = "Data: Initialize\nInitialize Core Data\nEvents: Register\nUI: Initialize\nUI: Front Panel State >> Open"  # Data: Initialize Initialize Core Data Events: Register UI: Initialize UI: Front Panel State >> Open
        # "Initialization Macro\n(This is called once, when the VI starts)"
        n95 = call <vilib>:"Add State(s) to Queue__JKI_lib_State_Machine.vi"("State(s) in Front (\"\")"=w322, "State(s) in (\"\")"=w326) -> ("States Out"=w325:string)  [unwired: 13 in]
      }
      frame "Macro: Exit" {
        # "Exit Macro\n(This is called once, when the VI exits)"
        n96 = Unbundle By Name(w334) -> ("Core.Close Panel on Exit?"=w333:bool)
        n97 = Select(t="UI: Front Panel State >> Close", s=w333, f="") -> (s? t:f=w330:string)
        n98 = call <vilib>:"Add State(s) to Queue__JKI_lib_State_Machine.vi"("State(s) in (\"\")"=w330, "State(s) at Back (\"\")"="Data: Cleanup\nEvents: Unregister\nExit") -> ("States Out"=w328:string)  [unwired: 13 in]
        n99 = call <vilib>:"Add State(s) to Queue__JKI_lib_State_Machine.vi"("State(s) in Front (\"\")"=w328, "State(s) in (\"\")"=w337) -> ("States Out"=w336:string)  [unwired: 13 in]
      }
      frame "---------- API ----------" {
        # "Do not put any code in this frame.\n(It is a separator no-op. This category is recommended to use for external API)"
      }
      frame "API: API1" {
        # "If you need to tell who triggered this state , use this string. If it's this case itself, this string is \"\"."
        # "Deal with the parameter if any"
        # "Connect this to return the response of your API"
        # "Copy/Rename this case for your own API"
      }
      frame "API: API2" {
        # "unpack HexStr  to Variant\nif complex parameter is needed."
        # "Copy/Rename this case for your own API"
        n100 = call "CSM - Convert HexStr to Data.vi"("HEX String"=w348) -> ()  [unwired: 7 in, 2 out]
        n101 = disable-structure shown="Disabled" {
          disable-tunnel: [w353 "API2 Response"] -> w347
          frame Disabled {
            # "pack variant to hexstr \nif complex response is needed."
            # "complex Response"
            n102 = call "CSM - Convert Data to HexStr.vi"() -> ("HEX String (0-9,A-F)"=w353:string)  [unwired: 9 in]
          }
          frame Enabled {
          }
        }
      }
      frame "---------- DoSth ----------" {
        # "Template Separator\n(You can make a copy of, or modify, this frame)"
        n103 = call <vilib>:"Add State(s) to Queue__JKI_lib_State_Machine.vi"("State(s) in (\"\")"=w359) -> ("States Out"=w358:string)  [unwired: 14 in]
      }
      frame "DoSth: DoA" {
        # "Your code here.\n(You can make a copy of, or modify, this frame)"
        n104 = call <vilib>:"Add State(s) to Queue__JKI_lib_State_Machine.vi"("State(s) in (\"\")"=w365) -> ("States Out"=w364:string)  [unwired: 14 in]
      }
      frame "DoSth: DoB" {
        # "Your code here.\n(You can make a copy of, or modify, this frame)"
        n105 = call <vilib>:"Add State(s) to Queue__JKI_lib_State_Machine.vi"("State(s) in (\"\")"=w371) -> ("States Out"=w370:string)  [unwired: 14 in]
      }
      frame "Handler: Error Occurred" {
        n106 = Unbundle(w378) -> ("‘State"=w373:string)  [unwired: 2 out]
        n107 = call "CSM - Convert Argument to Error.vi"("Argument"=w381) -> ("Error"=w372:errorcluster)  [unwired: 4 in]
        n108 = Unbundle By Name(w372) -> ("source"=w380:string)
        n109 = Concatenate Strings("From:" ("string"), w379) -> (w377:string)
        n110 = Concatenate Strings("Because:" ("string"), w373) -> (w376:string)
        n111 = Two Button Dialog(message=w380, 1:w376, 2:w377) -> ()  [unwired: 1 out]
      }
    }
  }
  n112 = while "JKI State Machine++ 2023" {
    shift-right: [w401] -> _
    shift-left: _ -> [w400]
    shift-right: [w404] -> _
    shift-left: _ -> [w398]
    shift-right: [w403] -> _
    shift-left: w1 -> [w405]
    tunnel: "Slave" ("Name(\"\" to use uuid)") -> [w394]
    shift-right: [w397] -> _
    shift-left: _ -> [w388]
    shift-right: [w396] -> _
    shift-left: _ -> [w395]
    stop <- w402 stop-if-true
    w399 = -1  # Timeout
    # "JKI-SM Copyright © 2018 JKI - http://jki.net/state-machine CSM Copyright ?2023 NEVSTOP https://github.com/NEVSTOP-LAB"
    # "copy this to add new state"
    # ">>"
    # "->"
    # "-@"
    # "copy this to create labels for wires"
    # "System_Label"
    n113 = call "Parse State Queue++.vi"("State Queue"=w405, "Name (\"\" to Use UUID)"=w394, "Response Arguments"=w388, "Previous Error"=w398, "Dequeue (1 ms)"=-1 ("Dequeue Timeout(0ms)")) -> ("Name Used"=w389:string, "Remaining States"=w406:string, "Current State"=w393:string, "Arguments"=w392:string, "Additional Information"=w391:T3, "Source CSM"=w390:string)  [unwired: 5 in]
    n114 = call "CSM - Internal State Debug Log History.vi"("State"=w393, "Arguments (\"\")"=w392, ">> Response Source Message >>"=w391, "Source (\"\")"=w390) -> ("Debug Log"=→"State History 2":string)  [unwired: 11 in]
    n115 = case shown="\"Target Timeout Error\"" w393 {
      selector: w393 -> [_ _ _ w422 _ _ _ _ _ _ _ _ _ _ _ _ _ _ _ _ _ _ _ _ _ _ _ _ _ _ _ _ _]
      tunnel: w406 -> [w408 w413 w419 w426 w443 w453 w461 w473 w482 w486 w501 w507 w512 w520 w527 w532 w538 w542 w548 w553 w560 w572 w642 w648 w659 w662 w667 w673 w681 w688 w694 w700 w704]
      tunnel: w392 -> [_ _ _ _ _ w446 w457 w469 _ _ _ _ _ _ _ _ _ _ _ _ w555 w566 _ _ _ _ _ w670 _ _ _ _ _]
      tunnel: w400 -> [w409 w412 w416 w424 w441 w454 w459 w471 w481 w485 w494 w505 w509 _ w522 w529 w537 w541 w545 w551 w558 w568 w639 w645 w656 w661 w666 w672 w678 w685 w691 w697 w703]
      tunnel: [w407 w414 w417 w428 errorcluster {"status"=FALSE, "code"=0, "source"=""} ("error out") w455 w463 w475 w483 w487 w498 w504 w510 w517 w523 w530 w533 w540 w546 w550 w556 w569 w640 w646 w657 w663 w668 w674 w679 w686 w692 w698 errorcluster {"status"=TRUE, "code"=-1, "source"="simulate an error in slave"} ("error out")] -> w404
      tunnel: w398 -> [w407 w414 w417 w427 w433 w455 w462 w474 w483 w487 w498 w504 w510 w517 w524 w530 _ w543 w546 w550 w557 w570 w640 w646 w657 w663 w668 w674 w679 w686 w692 w698 _]
      tunnel: [w408 w413 w418 w425 w435 w452 w460 w472 w482 w486 w500 w506 w511 w519 w526 w531 w538 w542 w547 w552 w559 w571 w641 w647 w658 w662 w667 w673 w680 w687 w693 w699 w704] -> w403
      tunnel: [_ _ _ _ _ TRUE _ _ _ _ _ TRUE _ _ _ _ _ _ _ _ _ _ _ _ _ _ _ _ _ _ _ _ _] -> w402
      tunnel: [w409 w412 w416 w424 w441 w454 w459 w471 w481 w485 w499 w505 w509 w518 w522 w529 w537 w541 w545 w551 w558 w568 w639 w645 w656 w661 w666 w672 w678 w685 w691 w697 w703] -> w401
      tunnel: w399 -> [_ _ _ _ _ _ _ _ _ _ _ _ _ _ _ _ _ _ _ _ _ _ _ _ _ _ _ _ _ _ _ _ _]
      tunnel: w390 -> [_ _ _ _ _ _ _ _ _ _ _ _ _ _ _ _ _ _ _ _ _ _ _ _ _ _ _ _ _ _ _ _ _]
      tunnel: w391 -> [_ _ _ _ _ _ _ _ _ _ _ _ _ _ _ _ _ _ _ _ _ _ _ _ _ _ _ _ _ _ _ _ _]
      tunnel: [_ _ _ "" _ _ _ _ _ _ _ _ _ _ _ _ _ _ _ _ _ _ _ _ _ _ "API1 Response" w669 _ "DoA Finished" "DoB Finished" _ _] -> w397
      tunnel: [w410 w411 w415 w420 w439 w444 w456 w468 w480 w484 w488 w502 w508 w513 w521 w528 w536 w539 w544 w549 w554 w565 w638 w643 w649 w660 w665 w671 w677 w684 w690 w696 w702] -> w396
      tunnel: w395 -> [w410 w411 w415 w420 w439 w444 w456 w468 w480 w484 w488 w502 w508 w513 w521 w528 _ w539 w544 w549 w554 w565 w638 w643 w649 w660 w665 w671 w677 w684 w690 w696 w702]
      tunnel: w389 -> [_ _ _ _ _ _ _ _ _ _ _ _ _ _ _ _ w535 _ _ _ _ _ _ _ _ _ _ _ _ _ _ _ _]
      tunnel: w388 -> [_ _ _ _ _ _ _ _ _ _ _ _ _ _ _ _ _ _ _ _ _ _ _ _ _ _ _ _ _ _ _ _ _]
      frame "", "Idle" {
        # "executes when the state queue is empty"
      }
      frame "CSM Documentation" {
        # "CSM Documentation"
        # "State Syntax:\nStateCategory: State >> Argument @|-> CSMName\nLine Terminator: Line feed\n\nExample:\nUI: Help >> About @Main\nUI: Help >> About ->Main"
        # "Commenting:\nTo add a comment use \"//\" or \"#\" and all text to the right will be ignored\nCommenting Example:\nUI: Initialize // This initializes the UI\n# This whole line is a comment\n// Another comment line"
      }
      frame "---------- Core ----------" {
        # "Do not put any code in this frame.\n(it is a separator no-op)"
        n116 = call <vilib>:"Add State(s) to Queue__JKI_lib_State_Machine.vi"("State(s) in (\"\")"=w419) -> ("States Out"=w418:string)  [unwired: 14 in]
      }
      frame Default {
        w431 = 42 items=["No error", "Argument error", "Memory is full", "Out of zone", "End of file", "File already open", "Generic file I/O error", "File not found", "File permission error", "Disk is full", "Duplicate path", "Too many files open", "System feature not enabled", "Resource file not found", "Cannot add resource", "Resource not found", "Image not found", "Image memory error", "Pen does not exist", "Config type invalid", "Config token not found", "Config parse error", "Config memory error", "Bad external code format", "Bad external code offset", "External code not present", "Null window", "Destroy window error", "Null menu", "Print aborted", "Bad print record", "Print driver error", "Windows error during printing", "Memory error during printing", "Print dialog error", "Generic print error", "Invalid device refnum", "Device not found", "Device parameter error", "Device unit error", "Cannot open device", "Device call aborted", "Generic error", "Cancelled by user", "Object ID too low", "Object ID too high", "Object not in heap", "Unknown heap", "Unknown object (invalid DefProc)", "Unknown object (DefProc not in table)", "Message out of range", "Invalid (null) method", "Unknown message", "Manager call not supported", "Bad address", "Network operation in progress", "Network operation timed out", "Connection is busy", "Network attribute not supported", "Network error", "Address in use", "System out of memory", "Connection aborted", "Connection refused", "Not connected", "Already connected", "Connection closed", "Initialization error (interapplication manager)", "Bad occurrence", "Wait on unbound occurrence handler", "Occurrence queue overflow", "Datalog type conflict", "Unused", "Unrecognized type (interapplication manager)", "Memory corrupt", "Failed to make temporary DLL", "Old CIN version", "Drag socket not found", "Failed to load drop-object", "Failed to register OLE object", "Failed to release OLE object", "Format specifier type mismatch", "Unknown format specifier", "Too few format specifiers", "Too many format specifiers", "Scan failed", "Newer CIN version", "Error converting to variant", "Runtime menu error", "Password tampered", "Variant attribute not found", "Incompatible variant data type", "Event data is not available", "Event Store is not present", "Occurrence is not found", "Event Queue is not created", "Event info is not available", "Refnum passed is NULL", "Error retrieving Class GUID", "Error retrieving CoClass GUID", "Error retrieving TypeLib GUID.", "Bad built application magic bytes.", "Specific driver is different from the specific driver associated with the Logical Name.", "There is no session opened to the class driver.", "Max Error", "MAX - Error with config objects", "MAX - Error loading configuration", "MAX - Group not supported"]
        # "Do not delete, rename, or modify this frame.\n(this is used to capture unhandled states and typos)"
        # "Handle mistyped state name (developer tool)"
        n117 = Format Into String(format string="Software Exception: Unhandled State \"%s\"." ("message"), error in=w427, w422) -> (resulting string=w430:string, error out=w429:errorcluster)  [unwired: 1 in]
        n118 = call <vilib>:"Error Cluster From Error Code.vi"("show call chain? (False)"=TRUE, "error in (no error)"=w429, "error message (\"\")"=w430, "error code (0)"=w431) -> ("error out"=w428:errorcluster)  [unwired: 5 in]
        n119 = call <vilib>:"Add State(s) to Queue__JKI_lib_State_Machine.vi"("State(s) in (\"\")"=w426) -> ("States Out"=w425:string)  [unwired: 14 in]
      }
      frame "Error Handler" {
        # "Handle any errors here.\nYou can also output any states to clean-up after errors occur"
        # "Clear error"
        n120 = call "CSM - Convert Error to Argument.vi"("Error"=w433) -> ("Argument"=w437:string)  [unwired: 4 in]
        n121 = call <vilib>:"Build State String with Arguments__JKI_lib_State_Machine.vi"("Arguments (\"\")"=w437, "State"="Error Occured" ("Status with Arguments")) -> ("State with Arguments"=w434:string)  [unwired: 4 in]
        n122 = call <vilib>:"Add State(s) to Queue__JKI_lib_State_Machine.vi"("State(s) in Front (\"\")"="/* Post Error States", "State(s) in (\"\")"=w443) -> ("States Out"=w436:string)  [unwired: 13 in]
        n123 = call "CSM - Broadcast Status Change.vi"("Status With Arguments"=w434, "State Queue"=w436) -> ("Remaining States"=w435:string)  [unwired: 13 in]
      }
      frame "Critical Error" {
        w450 = 42 items=["No error", "Argument error", "Memory is full", "Out of zone", "End of file", "File already open", "Generic file I/O error", "File not found", "File permission error", "Disk is full", "Duplicate path", "Too many files open", "System feature not enabled", "Resource file not found", "Cannot add resource", "Resource not found", "Image not found", "Image memory error", "Pen does not exist", "Config type invalid", "Config token not found", "Config parse error", "Config memory error", "Bad external code format", "Bad external code offset", "External code not present", "Null window", "Destroy window error", "Null menu", "Print aborted", "Bad print record", "Print driver error", "Windows error during printing", "Memory error during printing", "Print dialog error", "Generic print error", "Invalid device refnum", "Device not found", "Device parameter error", "Device unit error", "Cannot open device", "Device call aborted", "Generic error", "Cancelled by user", "Object ID too low", "Object ID too high", "Object not in heap", "Unknown heap", "Unknown object (invalid DefProc)", "Unknown object (DefProc not in table)", "Message out of range", "Invalid (null) method", "Unknown message", "Manager call not supported", "Bad address", "Network operation in progress", "Network operation timed out", "Connection is busy", "Network attribute not supported", "Network error", "Address in use", "System out of memory", "Connection aborted", "Connection refused", "Not connected", "Already connected", "Connection closed", "Initialization error (interapplication manager)", "Bad occurrence", "Wait on unbound occurrence handler", "Occurrence queue overflow", "Datalog type conflict", "Unused", "Unrecognized type (interapplication manager)", "Memory corrupt", "Failed to make temporary DLL", "Old CIN version", "Drag socket not found", "Failed to load drop-object", "Failed to register OLE object", "Failed to release OLE object", "Format specifier type mismatch", "Unknown format specifier", "Too few format specifiers", "Too many format specifiers", "Scan failed", "Newer CIN version", "Error converting to variant", "Runtime menu error", "Password tampered", "Variant attribute not found", "Incompatible variant data type", "Event data is not available", "Event Store is not present", "Occurrence is not found", "Event Queue is not created", "Event info is not available", "Refnum passed is NULL", "Error retrieving Class GUID", "Error retrieving CoClass GUID", "Error retrieving TypeLib GUID.", "Bad built application magic bytes.", "Specific driver is different from the specific driver associated with the Logical Name.", "There is no session opened to the class driver.", "Max Error", "MAX - Error with config objects", "MAX - Error loading configuration", "MAX - Group not supported"]
        # "Handle critical error here.\nWhen any un-recoverable error occurs, CSM goes into this case."
        # "When Critical Error occurs, Stop the loop immediately. Do NOT change this unless you fully understand the impact."
        # "Handle mistyped state name (developer tool)"
        n124 = Format Into String(format string="Software Exception: Critical Error\"%s\"." ("message"), w446) -> (resulting string=w449:string, error out=w448:errorcluster)  [unwired: 2 in]
        n125 = call <vilib>:"Error Cluster From Error Code.vi"("show call chain? (False)"=TRUE, "error in (no error)"=w448, "error message (\"\")"=w449, "error code (0)"=w450) -> ()  [unwired: 5 in, 1 out]
        n126 = call <vilib>:"Add State(s) to Queue__JKI_lib_State_Machine.vi"("State(s) in (\"\")"=w453) -> ("States Out"=w452:string)  [unwired: 14 in]
      }
      frame "Target Timeout Error" {
        w466 = 42 items=["No error", "Argument error", "Memory is full", "Out of zone", "End of file", "File already open", "Generic file I/O error", "File not found", "File permission error", "Disk is full", "Duplicate path", "Too many files open", "System feature not enabled", "Resource file not found", "Cannot add resource", "Resource not found", "Image not found", "Image memory error", "Pen does not exist", "Config type invalid", "Config token not found", "Config parse error", "Config memory error", "Bad external code format", "Bad external code offset", "External code not present", "Null window", "Destroy window error", "Null menu", "Print aborted", "Bad print record", "Print driver error", "Windows error during printing", "Memory error during printing", "Print dialog error", "Generic print error", "Invalid device refnum", "Device not found", "Device parameter error", "Device unit error", "Cannot open device", "Device call aborted", "Generic error", "Cancelled by user", "Object ID too low", "Object ID too high", "Object not in heap", "Unknown heap", "Unknown object (invalid DefProc)", "Unknown object (DefProc not in table)", "Message out of range", "Invalid (null) method", "Unknown message", "Manager call not supported", "Bad address", "Network operation in progress", "Network operation timed out", "Connection is busy", "Network attribute not supported", "Network error", "Address in use", "System out of memory", "Connection aborted", "Connection refused", "Not connected", "Already connected", "Connection closed", "Initialization error (interapplication manager)", "Bad occurrence", "Wait on unbound occurrence handler", "Occurrence queue overflow", "Datalog type conflict", "Unused", "Unrecognized type (interapplication manager)", "Memory corrupt", "Failed to make temporary DLL", "Old CIN version", "Drag socket not found", "Failed to load drop-object", "Failed to register OLE object", "Failed to release OLE object", "Format specifier type mismatch", "Unknown format specifier", "Too few format specifiers", "Too many format specifiers", "Scan failed", "Newer CIN version", "Error converting to variant", "Runtime menu error", "Password tampered", "Variant attribute not found", "Incompatible variant data type", "Event data is not available", "Event Store is not present", "Occurrence is not found", "Event Queue is not created", "Event info is not available", "Refnum passed is NULL", "Error retrieving Class GUID", "Error retrieving CoClass GUID", "Error retrieving TypeLib GUID.", "Bad built application magic bytes.", "Specific driver is different from the specific driver associated with the Logical Name.", "There is no session opened to the class driver.", "Max Error", "MAX - Error with config objects", "MAX - Error loading configuration", "MAX - Group not supported"]
        # "Handle target timeout error here.\nWhen this CSM could not get the sync-call response in time, this CSM goes into this case."
        # "Handle mistyped state name (developer tool)"
        n127 = Format Into String(format string="Software Exception: Target could not finish the \"%s\" state in time." ("message"), error in=w462, w457) -> (resulting string=w465:string, error out=w464:errorcluster)  [unwired: 1 in]
        n128 = call <vilib>:"Error Cluster From Error Code.vi"("show call chain? (False)"=TRUE, "error in (no error)"=w464, "error message (\"\")"=w465, "error code (0)"=w466) -> ("error out"=w463:errorcluster)  [unwired: 5 in]
        n129 = call <vilib>:"Add State(s) to Queue__JKI_lib_State_Machine.vi"("State(s) in (\"\")"=w461) -> ("States Out"=w460:string)  [unwired: 14 in]
      }
      frame "Target Error" {
        w478 = 42 items=["No error", "Argument error", "Memory is full", "Out of zone", "End of file", "File already open", "Generic file I/O error", "File not found", "File permission error", "Disk is full", "Duplicate path", "Too many files open", "System feature not enabled", "Resource file not found", "Cannot add resource", "Resource not found", "Image not found", "Image memory error", "Pen does not exist", "Config type invalid", "Config token not found", "Config parse error", "Config memory error", "Bad external code format", "Bad external code offset", "External code not present", "Null window", "Destroy window error", "Null menu", "Print aborted", "Bad print record", "Print driver error", "Windows error during printing", "Memory error during printing", "Print dialog error", "Generic print error", "Invalid device refnum", "Device not found", "Device parameter error", "Device unit error", "Cannot open device", "Device call aborted", "Generic error", "Cancelled by user", "Object ID too low", "Object ID too high", "Object not in heap", "Unknown heap", "Unknown object (invalid DefProc)", "Unknown object (DefProc not in table)", "Message out of range", "Invalid (null) method", "Unknown message", "Manager call not supported", "Bad address", "Network operation in progress", "Network operation timed out", "Connection is busy", "Network attribute not supported", "Network error", "Address in use", "System out of memory", "Connection aborted", "Connection refused", "Not connected", "Already connected", "Connection closed", "Initialization error (interapplication manager)", "Bad occurrence", "Wait on unbound occurrence handler", "Occurrence queue overflow", "Datalog type conflict", "Unused", "Unrecognized type (interapplication manager)", "Memory corrupt", "Failed to make temporary DLL", "Old CIN version", "Drag socket not found", "Failed to load drop-object", "Failed to register OLE object", "Failed to release OLE object", "Format specifier type mismatch", "Unknown format specifier", "Too few format specifiers", "Too many format specifiers", "Scan failed", "Newer CIN version", "Error converting to variant", "Runtime menu error", "Password tampered", "Variant attribute not found", "Incompatible variant data type", "Event data is not available", "Event Store is not present", "Occurrence is not found", "Event Queue is not created", "Event info is not available", "Refnum passed is NULL", "Error retrieving Class GUID", "Error retrieving CoClass GUID", "Error retrieving TypeLib GUID.", "Bad built application magic bytes.", "Specific driver is different from the specific driver associated with the Logical Name.", "There is no session opened to the class driver.", "Max Error", "MAX - Error with config objects", "MAX - Error loading configuration", "MAX - Group not supported"]
        # "Handle target error here.\nWhen this CSM try to communicate with an un-existed CSM, this CSM goes into this case."
        # "Handle mistyped state name (developer tool)"
        n130 = Format Into String(format string="Software Exception: Target \"%s\" does not exists." ("message"), error in=w474, w469) -> (resulting string=w477:string, error out=w476:errorcluster)  [unwired: 1 in]
        n131 = call <vilib>:"Error Cluster From Error Code.vi"("show call chain? (False)"=TRUE, "error in (no error)"=w476, "error message (\"\")"=w477, "error code (0)"=w478) -> ("error out"=w475:errorcluster)  [unwired: 5 in]
        n132 = call <vilib>:"Add State(s) to Queue__JKI_lib_State_Machine.vi"("State(s) in (\"\")"=w473) -> ("States Out"=w472:string)  [unwired: 14 in]
      }
      frame "Async Response", "Response" {
        # "Handle Async-call Response (\"Async Response\" for ->)"
        # "Handle Sync-call Response (\"Response\" for @)"
        # "After Message is executed, CSM goes to this state for receive the response. \n    For Async Message(->), \"Async Response\" is used. This CSM will goes to \"Async Message Posted\" immediately and receive the \"Async Response\" after the callee finishes the message.\n    For Sync Message(@),  This CSM will wait until the message is done and immediately goes to \"Response\""
      }
      frame "Async Message Posted" {
        # "Handle post action for async message (->)."
        # "After Async Message is posted (->), CSM goes to this state for post-action. You can use Argument - State to tell which Async Message is called."
      }
      frame "Initialize Core Data" {
        # "Do not delete, rename, or modify this frame.\n(this is used to determine panel behavior on exit)"
        # "originally closed?"
        # "exe?"
        # "If panel starts closed or is an EXE, then close it when we exit"
        n133 = property class="VI"() -> ("FP.State"=w491:T1)  [unwired: 2 in, 2 out]
        n134 = property class="App"() -> ("App.Kind"=w497:T2)  [unwired: 2 in, 2 out]
        n135 = control-ref of="Current VI Reference"() -> (w492:refnum<vi>)
        n136 = Equal?(x=w491, y=T1."Closed" ("Front Panel Window:State")) -> (x = y?=w489:bool)
        n137 = Equal?(x=w497, y=T2."Run Time System" ("Application:Kind")) -> (x = y?=w495:bool)
        n138 = Or(x=w489, y=w495) -> (x .or. y?=w493:bool)
        n139 = Bundle By Name(cluster=w494, "Core.Current VI Reference"=w492, "Core.Close Panel on Exit?"=w493) -> (w499:T5)
        n140 = call <vilib>:"Add State(s) to Queue__JKI_lib_State_Machine.vi"("State(s) in (\"\")"=w501) -> ("States Out"=w500:string)  [unwired: 14 in]
      }
      frame "Exit" {
        # "Do not put any code in this frame.\n(No errors that occur here will be handled.)"
        n141 = call <vilib>:"Add State(s) to Queue__JKI_lib_State_Machine.vi"("State(s) in (\"\")"=w507) -> ("States Out"=w506:string)  [unwired: 14 in]
      }
      frame "---------- Data ----------" {
        # "Do not put any code in this frame.\n(It is a separator no-op. You can make a copy of this frame to create a new Data frame)"
        n142 = call <vilib>:"Add State(s) to Queue__JKI_lib_State_Machine.vi"("State(s) in (\"\")"=w512) -> ("States Out"=w511:string)  [unwired: 14 in]
      }
      frame "Data: Initialize" {
        w514 = T4 {"Current VI Reference"=refnum, "Close Panel on Exit?"=FALSE}  # Core
        w516 = TRUE  # Your Boolean data
        w515 = ""  # Your string data
        # "do not delete - used by framework"
        # "Expand Bundle to add new data elements to shift register data."
        # "Add new data here."
        # "Data names and types of shift register data are defined by this bundle."
        # "Initialize the shift-register data, here.\n(data names are defined by what you wire into the bundle function)"
        n143 = Bundle("Core"=w514, "Your Boolean data"=w516, "Your string data"=w515) -> (w518:T5)  [unwired: 1 in]
        n144 = call <vilib>:"Add State(s) to Queue__JKI_lib_State_Machine.vi"("State(s) in (\"\")"=w520) -> ("States Out"=w519:string)  [unwired: 14 in]
      }
      frame "Data: Cleanup" {
        # "Cleanup any data and references, here.\n(this is called automatically, by the Macro: Exit)"
        n145 = Unbundle By Name(w522) -> ("Core.Current VI Reference"=w525:refnum<vi>)
        n146 = Close Reference(reference=w525, error in (no error)=w524) -> (error out=w523:errorcluster)
        n147 = call <vilib>:"Add State(s) to Queue__JKI_lib_State_Machine.vi"("State(s) in (\"\")"=w527) -> ("States Out"=w526:string)  [unwired: 14 in]
      }
      frame "---------- Events ----------" {
        # "Do not put any code in this frame.\n(It is a separator no-op. You can make a copy of this frame to create a new UI frame)"
        n148 = call <vilib>:"Add State(s) to Queue__JKI_lib_State_Machine.vi"("State(s) in (\"\")"=w532) -> ("States Out"=w531:string)  [unwired: 14 in]
      }
      frame "Events: Register" {
        # "Register message event to break Waiting in Event structure."
        n149 = call "CSM - Get New State Notifier Event.vi"("Name (\"\" to Use UUID)"=w535) -> ("error out"=w533:errorcluster, "New State Notifier Event"=w534:refnum<user-event>)  [unwired: 9 in]
        n150 = register-events(w534) -> (reference out=w536:refnum<event-registration>)  [unwired: 2 in, 1 out]
      }
      frame "Events: Unregister" {
        n151 = Unregister For Events(event registration refnum=w539, error in=w543) -> (error out=w540:errorcluster)
      }
      frame "---------- UI ----------" {
        # "Do not put any code in this frame.\n(It is a separator no-op. You can make a copy of this frame to create a new UI frame)"
        n152 = call <vilib>:"Add State(s) to Queue__JKI_lib_State_Machine.vi"("State(s) in (\"\")"=w548) -> ("States Out"=w547:string)  [unwired: 14 in]
      }
      frame "UI: Initialize" {
        # "Initialize the User Interface, here.\n(this is called automatically, by the Macro: Init)"
        n153 = call <vilib>:"Add State(s) to Queue__JKI_lib_State_Machine.vi"("State(s) in (\"\")"=w553) -> ("States Out"=w552:string)  [unwired: 14 in]
      }
      frame "UI: Cursor Set" {
        # "Argument"
        # "Set and Unset Cursor Busy.\n(Usage: \"UI: Cursor Set >> Busy|Idle\")"
        n154 = case shown="\"Idle\", Default" w555 {
          tunnel: w557 -> [w562 w564]
          tunnel: [w561 w563] -> w556
          frame "Idle", Default {
            n155 = call <vilib>:"Unset Busy.vi"("error in (no error)"=w562) -> ("error out"=w561:errorcluster)  [unwired: 10 in]
          }
          frame "Busy" {
            n156 = call <vilib>:"Set Busy.vi"("error in (no error)"=w564) -> ("error out"=w563:errorcluster)  [unwired: 9 in, 1 out]
          }
        }
        n157 = call <vilib>:"Add State(s) to Queue__JKI_lib_State_Machine.vi"("State(s) in (\"\")"=w560) -> ("States Out"=w559:string)  [unwired: 14 in]
      }
      frame "UI: Front Panel State" {
        # "Argument"
        # "Set Front Panel Open or Closed\n(Usage: \"UI: Front Panel State >> Open|Close\")"
        n158 = Unbundle By Name(w568) -> ("Core.Current VI Reference"=w567:refnum<vi>)
        n159 = case shown="\"Minimize\", \"Minimized\"" w566 {
          tunnel: w570 -> [w578 w593 w604 w617 w630]
          tunnel: [w580 w594 w606 w619 w632] -> w569
          tunnel: w567 -> [w579 w591 w605 w618 w631]
          frame "Open", "Standard", Default {
            w573 = T1."Standard" ("State")
            n160 = property class="VI"(reference=w579, error in=w578) -> (reference out=w576:refnum<vi>, error out=w577:errorcluster, "FP.State"=w575:T1)
            n161 = Not Equal?(x=w575, y=w573) -> (x != y?=w574:bool)
            n162 = case shown="True" w574 {
              tunnel: [w584 w586] -> w580
              tunnel: w577 -> [w583 w586]
              tunnel: w576 -> [w582 _]
              tunnel: w573 -> [w581 _]
              frame True {
                n163 = invoke class="VI" method="FP.Open"(reference=w582, error in=w583, "Activate"=TRUE, "State"=w581) -> (error out=w584:errorcluster)  [unwired: 1 in, 4 out]
              }
              frame False {
              }
            }
          }
          frame "Close", "Closed" {
            n164 = property class="VI"(reference=w591, error in=w593) -> (reference out=w590:refnum<vi>, error out=w592:errorcluster, "FP.State"=w588:T1)
            n165 = Not Equal?(x=w588, y=T1."Closed" ("Front Panel Window:State")) -> (x != y?=w587:bool)
            n166 = case shown="True" w587 {
              tunnel: [w595 w598] -> w594
              tunnel: w592 -> [w595 w597]
              tunnel: w590 -> [_ w596]
              frame False {
              }
              frame True {
                n167 = invoke class="VI" method="FP.Close"(reference=w596, error in=w597) -> (error out=w598:errorcluster)  [unwired: 1 in, 2 out]
              }
            }
          }
          frame "Hidden", "Hide" {
            w599 = T1."Hidden" ("State")
            n168 = property class="VI"(reference=w605, error in=w604) -> (reference out=w602:refnum<vi>, error out=w603:errorcluster, "FP.State"=w601:T1)
            n169 = Not Equal?(x=w601, y=w599) -> (x != y?=w600:bool)
            n170 = case shown="True" w600 {
              tunnel: [w610 w611] -> w606
              tunnel: w603 -> [w609 w611]
              tunnel: w602 -> [w608 _]
              tunnel: w599 -> [w607 _]
              frame True {
                n171 = invoke class="VI" method="FP.Open"(reference=w608, error in=w609, "State"=w607) -> (error out=w610:errorcluster)  [unwired: 2 in, 4 out]
              }
              frame False {
              }
            }
          }
          frame "Minimize", "Minimized" {
            w612 = T1."Minimized" ("State")
            n172 = property class="VI"(reference=w618, error in=w617) -> (reference out=w615:refnum<vi>, error out=w616:errorcluster, "FP.State"=w614:T1)
            n173 = Not Equal?(x=w614, y=w612) -> (x != y?=w613:bool)
            n174 = case shown="True" w613 {
              tunnel: [w623 w624] -> w619
              tunnel: w616 -> [w622 w624]
              tunnel: w615 -> [w621 _]
              tunnel: w612 -> [w620 _]
              frame True {
                n175 = invoke class="VI" method="FP.Open"(reference=w621, error in=w622, "State"=w620) -> (error out=w623:errorcluster)  [unwired: 2 in, 4 out]
              }
              frame False {
              }
            }
          }
          frame "Maximize", "Maximized" {
            w625 = T1."Maximized" ("State")
            n176 = property class="VI"(reference=w631, error in=w630) -> (reference out=w628:refnum<vi>, error out=w629:errorcluster, "FP.State"=w627:T1)
            n177 = Not Equal?(x=w627, y=w625) -> (x != y?=w626:bool)
            n178 = case shown="True" w626 {
              tunnel: [w636 w637] -> w632
              tunnel: w629 -> [w635 w637]
              tunnel: w628 -> [w634 _]
              tunnel: w625 -> [w633 _]
              frame True {
                n179 = invoke class="VI" method="FP.Open"(reference=w634, error in=w635, "State"=w633) -> (error out=w636:errorcluster)  [unwired: 2 in, 4 out]
              }
              frame False {
              }
            }
          }
        }
        n180 = call <vilib>:"Add State(s) to Queue__JKI_lib_State_Machine.vi"("State(s) in (\"\")"=w572) -> ("States Out"=w571:string)  [unwired: 14 in]
      }
      frame "---------- Macro ----------" {
        # "Do not put any code in this frame.\n(It is a separator no-op. You can make a copy of this frame to create a new Macro frame)"
        n181 = call <vilib>:"Add State(s) to Queue__JKI_lib_State_Machine.vi"("State(s) in (\"\")"=w642) -> ("States Out"=w641:string)  [unwired: 14 in]
      }
      frame "Macro: Initialize" {
        w644 = "Data: Initialize\nInitialize Core Data\nEvents: Register\nUI: Initialize\nUI: Front Panel State >> Open"  # Data: Initialize Initialize Core Data Events: Register UI: Initialize UI: Front Panel State >> Open
        # "Initialization Macro\n(This is called once, when the VI starts)"
        n182 = call <vilib>:"Add State(s) to Queue__JKI_lib_State_Machine.vi"("State(s) in Front (\"\")"=w644, "State(s) in (\"\")"=w648) -> ("States Out"=w647:string)  [unwired: 13 in]
      }
      frame "Macro: Exit" {
        # "Exit Macro\n(This is called once, when the VI exits)"
        n183 = Unbundle By Name(w656) -> ("Core.Close Panel on Exit?"=w655:bool)
        n184 = Select(t="UI: Front Panel State >> Close", s=w655, f="") -> (s? t:f=w652:string)
        n185 = call <vilib>:"Add State(s) to Queue__JKI_lib_State_Machine.vi"("State(s) in (\"\")"=w652, "State(s) at Back (\"\")"="Data: Cleanup\nEvents: Unregister\nExit") -> ("States Out"=w650:string)  [unwired: 13 in]
        n186 = call <vilib>:"Add State(s) to Queue__JKI_lib_State_Machine.vi"("State(s) in Front (\"\")"=w650, "State(s) in (\"\")"=w659) -> ("States Out"=w658:string)  [unwired: 13 in]
      }
      frame "---------- API ----------" {
        # "Do not put any code in this frame.\n(It is a separator no-op. This category is recommended to use for external API)"
      }
      frame "API: API1" {
        # "If you need to tell who triggered this state , use this string. If it's this case itself, this string is \"\"."
        # "Deal with the parameter if any"
        # "Connect this to return the response of your API"
        # "Copy/Rename this case for your own API"
      }
      frame "API: API2" {
        # "unpack HexStr  to Variant\nif complex parameter is needed."
        # "Copy/Rename this case for your own API"
        n187 = call "CSM - Convert HexStr to Data.vi"("HEX String"=w670) -> ()  [unwired: 7 in, 2 out]
        n188 = disable-structure shown="Disabled" {
          disable-tunnel: [w675 "API2 Response"] -> w669
          frame Disabled {
            # "pack variant to hexstr \nif complex response is needed."
            # "complex Response"
            n189 = call "CSM - Convert Data to HexStr.vi"() -> ("HEX String (0-9,A-F)"=w675:string)  [unwired: 9 in]
          }
          frame Enabled {
          }
        }
      }
      frame "---------- DoSth ----------" {
        # "Template Separator\n(You can make a copy of, or modify, this frame)"
        n190 = call <vilib>:"Add State(s) to Queue__JKI_lib_State_Machine.vi"("State(s) in (\"\")"=w681) -> ("States Out"=w680:string)  [unwired: 14 in]
      }
      frame "DoSth: DoA" {
        # "Your code here.\n(You can make a copy of, or modify, this frame)"
        n191 = call <vilib>:"Add State(s) to Queue__JKI_lib_State_Machine.vi"("State(s) in Front (\"\")"="Slave Status Changed -> <all>" ("State(s) in Front (\"\")"), "State(s) in (\"\")"=w688) -> ("States Out"=w687:string)  [unwired: 13 in]
      }
      frame "DoSth: DoB" {
        # "Your code here.\n(You can make a copy of, or modify, this frame)"
        n192 = call <vilib>:"Add State(s) to Queue__JKI_lib_State_Machine.vi"("State(s) in (\"\")"=w694) -> ("States Out"=w693:string)  [unwired: 14 in]
      }
      frame "Status Change" {
        # "Your code here.\n(You can make a copy of, or modify, this frame)"
        n193 = call "CSM - Broadcast Status Change.vi"("Status With Arguments"="Slave Status Changed" ("State(s) in Front (\"\")"), "State Queue"=w700) -> ("Remaining States"=w699:string)  [unwired: 13 in]
      }
      frame "simulate an error" {
      }
    }
  }
